vi "PQinsert.vi"(5 "values":string[](array[string]), 6 "columns":string[](array[string]), 7 "table":string, 8 "conn":u32) -> (1 "PQresultErrorMessage":string, 2 "PQresultStatus":T1(ring), 3 "conn_out":u32)   [LabVIEW 2019, in "libpqutility.lvlib"]
doc: "Function to INSERT Values into named Columns of named Table. conn is the reference to database connection. See PostgreSQL c-lib doku for further information."
uses:
  libpqutility.lvlib
  colArrayToCommaString.vi
  libpqlv/libpqlv.lvlib
panel:
  out "INSERTstring":string
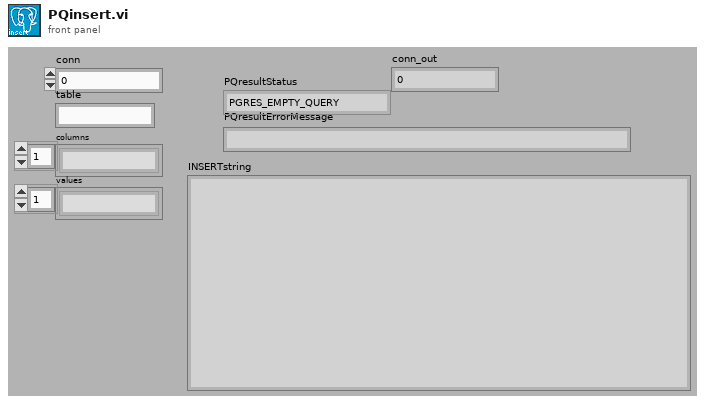
[diagram p1: front panel]
types:
  T1 = enum16{"PGRES_EMPTY_QUERY", "PGRES_COMMAND_OK", "PGRES_TUPLES_OK", "PGRES_COPY_OUT", "PGRES_COPY_IN", "PGRES_BAD_RESPONSE", "PGRES_NONFATAL_ERROR", "PGRES_FATAL_ERROR"}
  T2 = enum32{"PGRES_EMPTY_QUERY", "PGRES_COMMAND_OK", "PGRES_TUPLES_OK", "PGRES_COPY_OUT", "PGRES_COPY_IN", "PGRES_BAD_RESPONSE", "PGRES_NONFATAL_ERROR", "PGRES_FATAL_ERROR"}
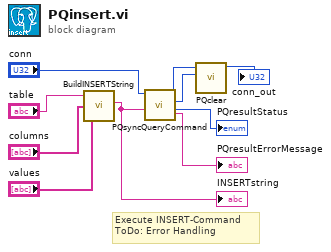
[diagram p0: block diagram]
diagram:
  # "Execute INSERT-Command\nToDo: Error Handling"
  n1 = call "BuildINSERTString.vi"("values"="values", "columns"="columns", "table"="table") -> ("INSERTstring"=w3:string)  [unwired: 5 in]
  "INSERTstring" <- w3
  n2 = call "PQsyncQueryCommand.vi"("query"=w3, "conn"="conn") -> ("PQresultStatus"=→"PQresultStatus":T2, "PGresult"=w5:u32, "conn out"=w2:u32, "PQresultErrorMessage"=→"PQresultErrorMessage":string)  [unwired: 5 in, 1 out]
  n3 = call "PQclear.vi"("res"=w5, "conn"=w2) -> ("conn_out"=→"conn_out":u32)  [unwired: 8 in, 1 out]
